vi "Configure 2 Input Logic Operation Inputs.vi"(6 "Selected Function (1)":u8=1 min=1 max=24, 7 "Unit Address (1)":u8=1, 8 "error in (no error)":errorcluster, 9 "Input 2 (0)":i32, 10 "Input 1 (0)":i32, 11 "VISA resource name":refnum<visa-resource-name>) -> (0 "error out":errorcluster, 3 "VISA resource name out":refnum<visa-resource-name>)   [LabVIEW 2014, in "Eurotherm 35xx Series.lvlib"]
doc: "This VI sets the input values for the Two Input Logic Operation Function."
uses:
  <instrlib>/Eurotherm 35xx Series/Eurotherm 35xx Series.lvlib
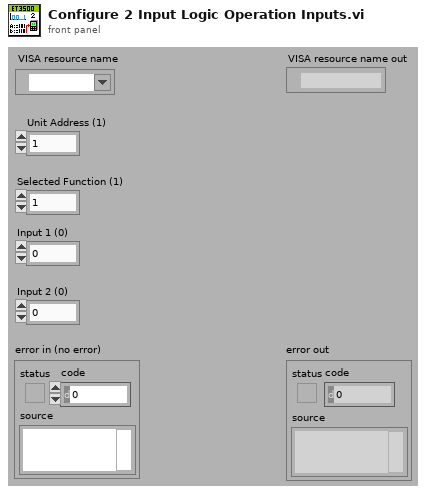
[diagram p1: front panel]
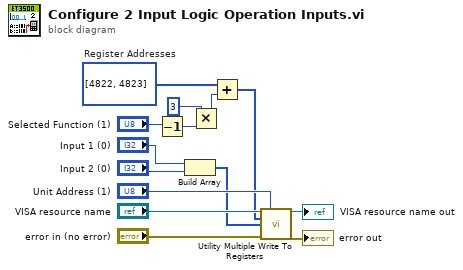
[diagram p0: block diagram]
diagram:
  w2 = i32[] [4822, 4823]  # Register Addresses
  n1 = Decrement(x="Selected Function (1)") -> (x-1=w5:u8)
  n2 = Build Array("Input 1 (0)", "Input 2 (0)") -> (w7:i32[])
  n3 = Multiply(x=u8 3, y=w5) -> (x*y=w3:u8)
  n4 = Add(x=w2, y=w3) -> (x+y=w1:i32[])
  n5 = call <instrlib>:"Utility Multiple Write To Registers.vi"("VISA resource name"="VISA resource name", "Unit Address (1)"="Unit Address (1)", "Registers Addresses (0)"=w1, "Data (0)"=w7, "error in (no error)"="error in (no error)") -> ("VISA resource name out"=→"VISA resource name out":refnum<visa-resource-name>, "error out"=→"error out":errorcluster)  [unwired: 9 in]
